vi "Close.vi"(8 "error in (no error)":errorcluster, 11 "refnum in":refnum<visa-resource-name>) -> (0 "error out":errorcluster)   [LabVIEW 2020, in "Korad KA3305P.lvlib"]
uses:
  Korad KA3305P.lvlib
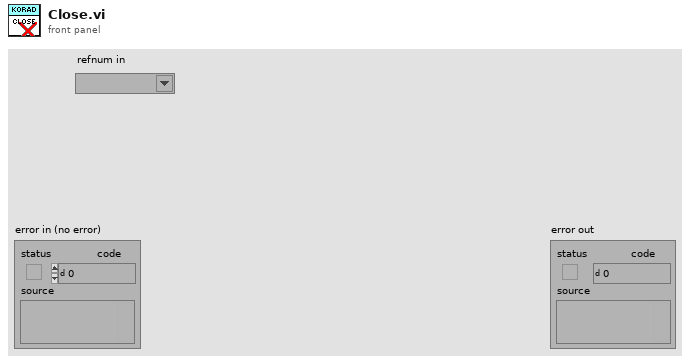
[diagram p1: front panel]
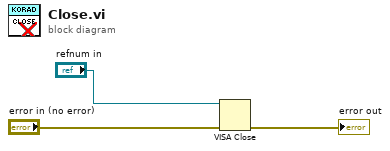
[diagram p0: block diagram]
diagram:
  n1 = VISA Close(VISA resource name="refnum in", error in (no error)="error in (no error)") -> (error out=→"error out":errorcluster)
